vi "Create LVProjects Error Message.vi"(8 "error in":errorcluster) -> (0 "error out":errorcluster)   [LabVIEW 2026, in "NIVS_CDEW_MetaDataObj.lvclass"]
uses:
  NIVS_CDEW_MetaDataObj.lvclass
  NIVS_CDEW_MetaDataObj.lvclass/NIVS_CDEW_MetaDataObj.ctl
  Types/Errors.ctl
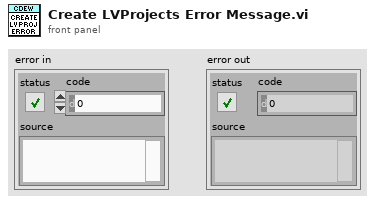
[diagram p1: front panel]
types:
  T1 = typedef "NIVS_CDEW_MetaDataObj.lvclass/Errors.ctl" = i32
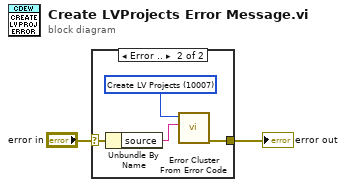
[diagram p0: block diagram]
diagram:
  n1 = case shown="Error .." "error in" {
    selector: "error in" -> [w3 w5]
    tunnel: [w3 w7] -> w1
    frame No Error {
    }
    frame Error {
      w6 = T1 10007 items=["Invalid XML File"=10001, "Missing File/Folder"=10002, "Duplicate CD in Root"=10003, "API Auto Gen"=10004, "Build APIs"=10005, "Clusters Auto Gen"=10006, "Create LV Projects"=10007] ("Errors")
      n2 = Unbundle By Name(w5) -> ("source"=w4:string)
      n3 = call <vilib>:"Error Cluster From Error Code.vi"("error message (\"\")"=w4, "error code (0)"=w6) -> ("error out"=w7:errorcluster)  [unwired: 7 in]
    }
  }
  "error out" <- w1
